vi "Sum_2D_array_to_1D.vi"(4 "Cols/rows?":bool, 5 "Array in":dbl[][](array[numeric])) -> (1 "Array average":dbl[](array[numeric]), 2 "Array summed":dbl[](array[numeric]))   [LabVIEW 2017]
panel:
  out "Plot result array":dbl[](graph)
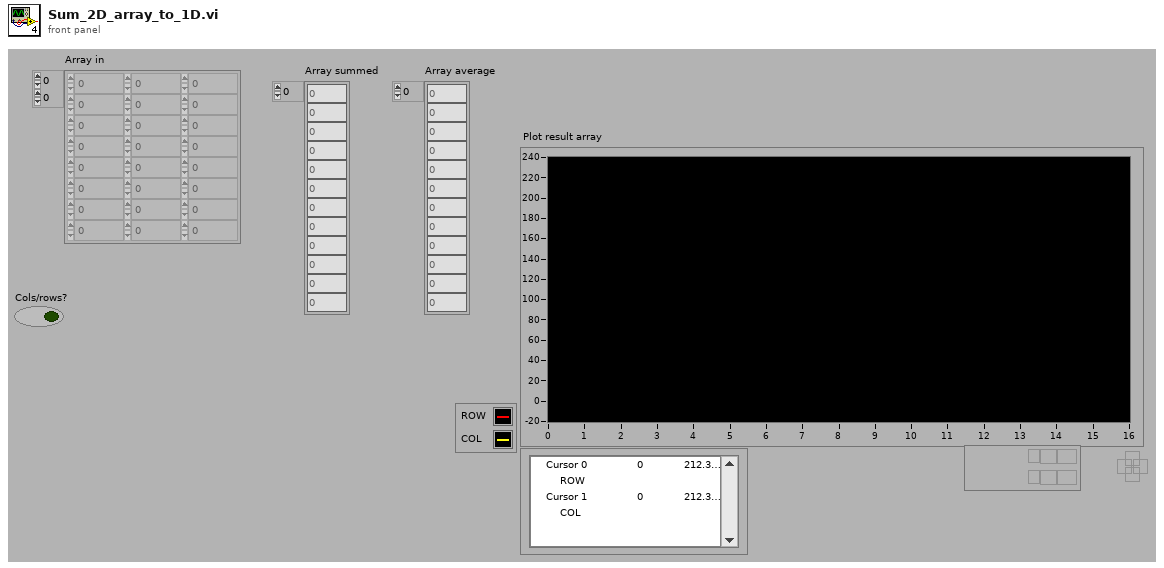
[diagram p1: front panel]
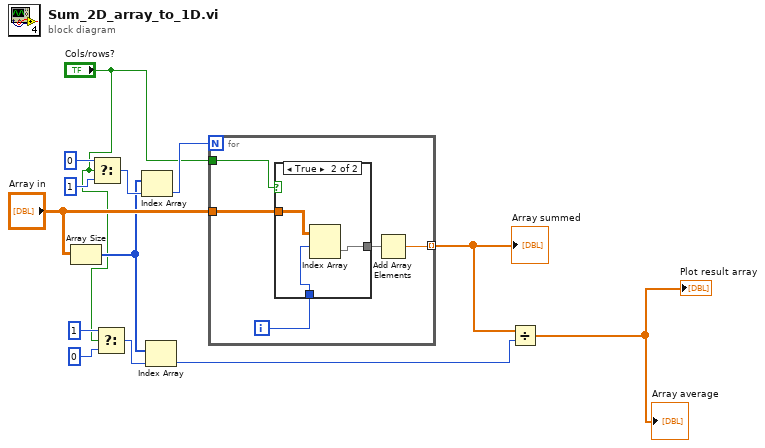
[diagram p0: block diagram]
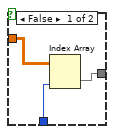
[diagram p2: hidden frame]
diagram:
  n1 = Array Size(array="Array in") -> (size(s)=w5:i32[])
  n2 = Select(t=i8 0, s="Cols/rows?", f=i8 1 ("t")) -> (s? t:f=w12:i8)
  n3 = Select(t=i8 1, s="Cols/rows?", f=i8 0 ("t")) -> (s? t:f=w6:i8)
  n4 = Index Array(array=w5, index=w12) -> (element=w9:i32)
  n5 = Index Array(array=w5, index=w6) -> (element=w4:i32)
  n6 = for {
    N: w9 -> [_]
    tunnel: [w18] -> w2 mode=indexing
    tunnel: "Array in" -> [w17]
    tunnel: "Cols/rows?" -> [w15]
    i -> [w14]
    n7 = case shown="True" w15 {
      tunnel: w17 -> [w20 w24]
      tunnel: [w21 w23] -> w16
      tunnel: w14 -> [w19 w22]
      frame False {
        n8 = Index Array(array=w20, index (col)=w19) -> (element=w21:dbl[])  [unwired: 1 in]
      }
      frame True {
        n9 = Index Array(array=w24, index (row)=w22) -> (element=w23:dbl[])  [unwired: 1 in]
      }
    }
    n10 = Add Array Elements(numeric array=w16) -> (sum=w18:dbl)
  }
  "Array summed" <- w2
  n11 = Divide(x=w2, y=w4) -> (x/y=→"Plot result array" →"Array average":dbl[])
